vi "Reset.vi"(8 "Error In":errorcluster, 10 "Reset Target":T7, 11 "LINX Resource":T1) -> (0 "Error Out":errorcluster, 3 "LINX Resource out":T1)   [LabVIEW 2019, in "LINXx.lvlib"]
uses:
  LINXx.lvlib
  Reset Target.ctl
  <vilib>/MakerHub/LINX/Private/Type Defs/LINX Ref.ctl
  <vilib>/MakerHub/LINX/Private/Type Defs/Platform.ctl
  <vilib>/MakerHub/LINX/Private/Type Defs/Interface.ctl
  <vilib>/MakerHub/LINX/Private/Device/Type Defs/LINX Device Config.ctl
  <vilib>/MakerHub/LINX/Private/Device/Type Defs/TCP Config.ctl
  <vilib>/MakerHub/LINX/Private/Device/Type Defs/Channels.ctl
  <vilib>/MakerHub/LINX/LMH-LINX.lvlib
  <vilib>/MakerHub/LINX/Private/Device/Device.lvlib
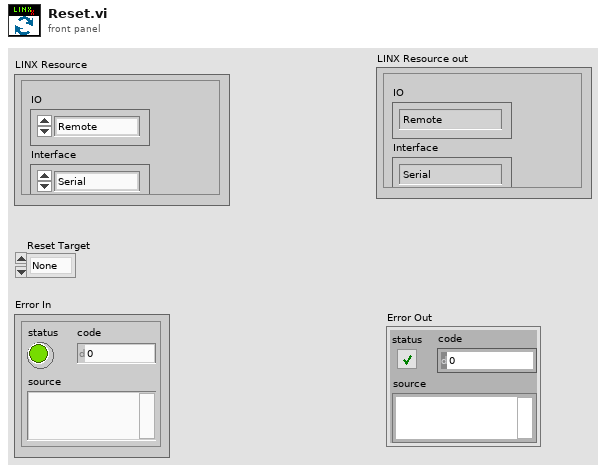
[diagram p1: front panel]
types:
  T1 = typedef "LMH-LINX.lvlib/LINX Ref.ctl" = cluster{"IO":T2, "Interface":T3, "LINX Device Config":T4}
  T2 = typedef "LMH-LINX.lvlib/Platform.ctl" = enum16{"Remote", "Local"}
  T3 = typedef "LMH-LINX.lvlib/Interface.ctl" = enum16{"Serial", "TCP"}
  T4 = typedef "LMH-LINX.lvlib/Device.lvlib/LINX Device Config.ctl" = cluster{"Interface":T3, "COM Port":refnum<visa-resource-name>, "TCP Configuration":T5, "Device Family":u8, "Device ID":u8, "Device Name":string, "TCP Ref":refnum<k5>, "Channels":T6}
  T5 = typedef "LMH-LINX.lvlib/Device.lvlib/TCP Config.ctl" = cluster{"IP Address":string, "Port":u16}
  T6 = typedef "LMH-LINX.lvlib/Channels.ctl" = cluster{"DI":u8[], "DO":u8[], "AI":u8[], "AO":u8[], "PWM":u8[], "QE":u8[], "UART":u8[], "I2C 2":u8[], "SPI":u8[], "CAN":u8[], "Servo":u8[], "AI Ref (V)":dbl, "AI Resolution (Bits)":u8, "AO Ref (V)":dbl, "AO Resolution (Bits)":u8}
  T7 = typedef "LINXx.lvlib/Reset Target.ctl" = enum16{"None", "Serial", "TCP", "Board"}
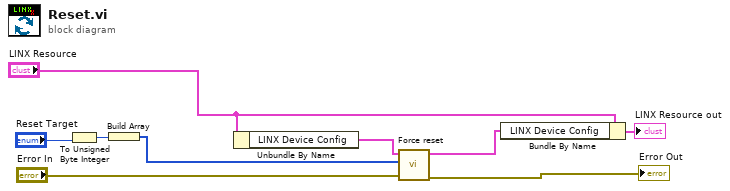
[diagram p0: block diagram]
diagram:
  n1 = To Unsigned Byte Integer(number="Reset Target") -> (unsigned 8bit integer=w8:u8)
  n2 = Build Array(w8) -> (w6:u8[])
  n3 = Unbundle By Name("LINX Resource") -> ("LINX Device Config"=w7:T4)
  n4 = call "Force reset.vi"("Error In"="Error In", "Reset Target"=w6, "LINX Device Config"=w7) -> ("Error Out"=→"Error Out":errorcluster, "Dup LINX Device Config"=w3:T4)  [unwired: 7 in]
  n5 = Bundle By Name(cluster="LINX Resource", "LINX Device Config"=w3) -> (→"LINX Resource out":T1)
